vi "Measure.vi"(8 "error in (no error)":errorcluster, 9 "measurement configuration":variant, 10 "measure call context in":refnum<class "Measure Call Context.lvclass">, 11 "measurement plugin in":refnum<class "FPT Intermodulation.lvclass">) -> (0 "error out":errorcluster, 1 "measurement results":variant, 2 "measure call context out":refnum<class "Measure Call Context.lvclass">, 3 "measurement plugin out":refnum<class "FPT Intermodulation.lvclass">)   [LabVIEW 2023, in "FPT Intermodulation.lvclass"]
uses:
  FPT Intermodulation.lvclass
  <vilib>/Plug-In SDKs/Measurements/Measure Call Context/Measure Call Context.lvclass
  Measurement Configuration.ctl
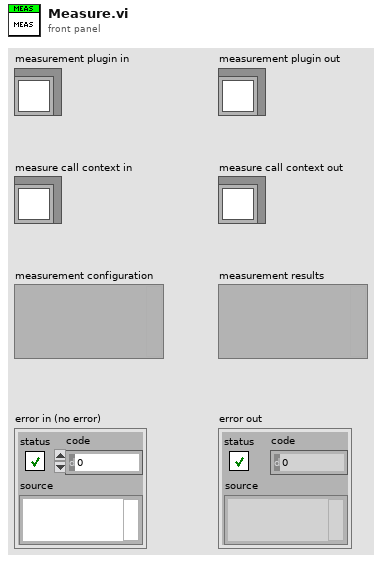
[diagram p1: front panel]
types:
  T1 = typedef "FPT Intermodulation.lvclass/Measurement Configuration.ctl" = cluster{"Automation Test":bool, "Power sequencing file path":string, "RFSG name":string, "RFSG port":string, "RFSG attenuation mode":enum32{"<None>", "Constant Attenuation", "s2p File"}, "RFSG external attenuation (dB)":dbl, "RFSG s-parameters orientation":enum32{"Port1 Towards DUT", "Port2 Towards DUT"}, "RFSG s2p file path":string, "RFmx name":string, "RFmx port":string, "RFmx attenuation mode":enum32{"<None>", "Constant Attenuation", "s2p File"}, "RFmx external attenuation (dB)":dbl, "RFmx s-parameters orientation":enum32{"Port1 Towards DUT", "Port2 Towards DUT"}, "RFmx s2p file path":string, "RFmx Reference Level (dBm)":dbl, "RFSG Generation IQ Rate (S/s)":dbl, "Target Pout Per Tone (dBm)":dbl, "Start Pin Per Tone (dBm)":dbl, "Start Center Frequency (Hz)":dbl, "Start Tone Spacing (Hz)":dbl, "IM_Sweep Mode":enum32{"Power", "Frequency", "Tone Spacing"}, "Sweep Delay (ms)":u32, "Power Sweep End":dbl, "Power Sweep Step":dbl, "Frequency Sweep End":dbl, "Frequency Sweep Step":dbl, "Tone Spacing Sweep End":dbl, "Tone Spacing Sweep Step":dbl, "Power sequencing file validity check":bool}
  T2 = typedef "FPT Intermodulation.lvclass/Measurement Results.ctl" = cluster{"Status":string, "Typical OIP3 (dBm)":dbl, "TS_Fundamental (dBm)":dbl[][], "TS_IMD (dBm)":dbl[][], "TS_TOI (dBm)":dbl[][], "TS_DUT Gain (dBm)":dbl[][], "TS_Fundamental Slope (dBm)":dbl[][], "TS_Intermodulation Slope (dBm)":dbl[][], "Final Target Pout (dBm)":dbl}
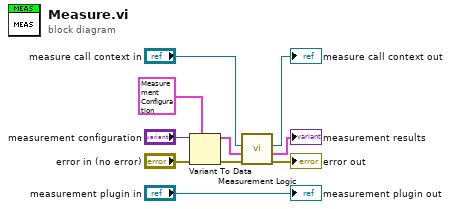
[diagram p0: block diagram]
diagram:
  n1 = Variant To Data(error in="error in (no error)", type=T1 {"Automation Test"=FALSE, "Power sequencing file path"="Lorem ipsum dolor sit", "RFSG name"="5842_0", "RFSG port"="", "RFSG attenuation mode"=enum."s2p File", "RFSG external attenuation (dB)"=1.2, "RFSG s-parameters orientation"=enum."Port1 Towards DUT", "RFSG s2p file path"="", "RFmx name"="5842_0", "RFmx port"="Lorem ipsum dolor sit", "RFmx attenuation mode"=enum."Constant Attenuation", "RFmx external attenuation (dB)"=1.0, "RFmx s-parameters orientation"=enum."Port2 Towards DUT", "RFmx s2p file path"="", "RFmx Reference Level (dBm)"=10.0, "RFSG Generation IQ Rate (S/s)"=1250000000.0, "Target Pout Per Tone (dBm)"=10.0, "Start Pin Per Tone (dBm)"=10.0, "Start Center Frequency (Hz)"=10.0, "Start Tone Spacing (Hz)"=10.0, "IM_Sweep Mode"=enum."Power", "Sweep Delay (ms)"=10, "Power Sweep End"=10.0, "Power Sweep Step"=10.0, "Frequency Sweep End"=-4.0, "Frequency Sweep Step"=1.0, "Tone Spacing Sweep End"=-4.0, "Tone Spacing Sweep Step"=1.0, "Power sequencing file validity check"=FALSE} ("measurement configuration"), Variant="measurement configuration") -> (data=w1:T1, error out=w7:errorcluster)
  n2 = call "Measurement Logic.vi"("error in"=w7, "measurement configuration"=w1, "measure call context in"="measure call context in") -> ("error out"=→"error out":errorcluster, "measurement results"=→"measurement results":T2, "measure call context out"=→"measure call context out":refnum<class "Measure Call Context.lvclass">)  [unwired: 6 in]
  "measurement plugin out" <- "measurement plugin in"
